vi "Write Control Width.vi"(8 "error in":errorcluster, 10 "Width":u32, 11 "Control in":refnum<vi>) -> (0 "error out":errorcluster, 3 "Control":refnum<vi>)   [LabVIEW 2020, in "VolatusGUIEditorCore.lvlib"]
uses:
  VolatusGUIEditorCore.lvlib
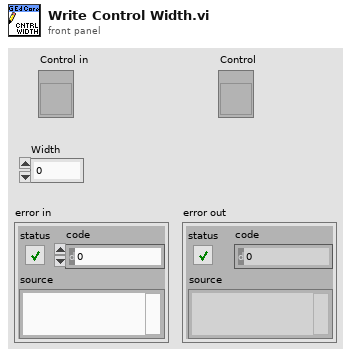
[diagram p1: front panel]
types:
  T1 = typedef "LVBoundsTypeDef.ctl" = cluster{"Width":u32, "Height":u32}
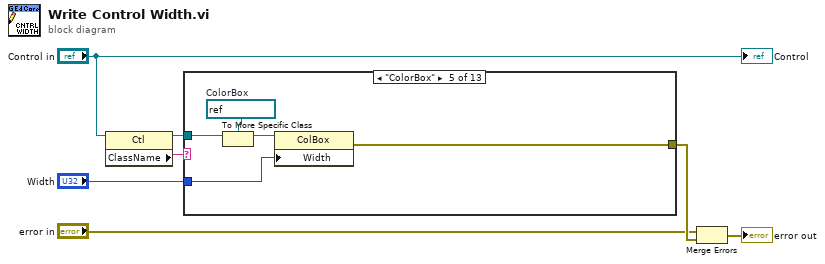
[diagram p0: block diagram]
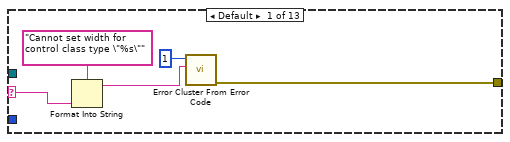
[diagram p2: hidden frame]
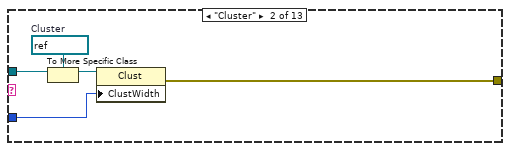
[diagram p3: hidden frame]
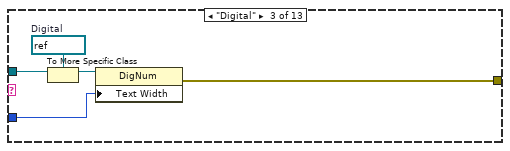
[diagram p4: hidden frame]
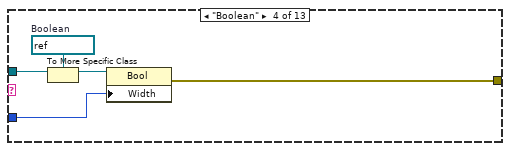
[diagram p5: hidden frame]
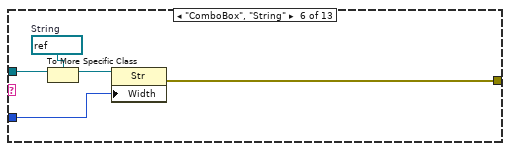
[diagram p6: hidden frame]
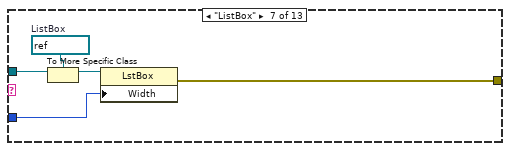
[diagram p7: hidden frame]
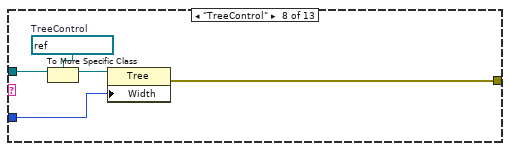
[diagram p8: hidden frame]
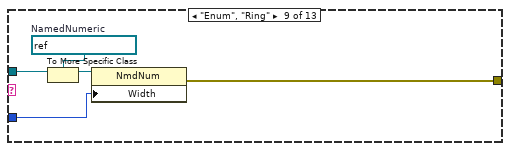
[diagram p9: hidden frame]
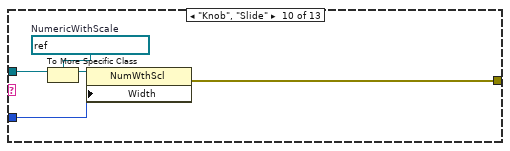
[diagram p10: hidden frame]
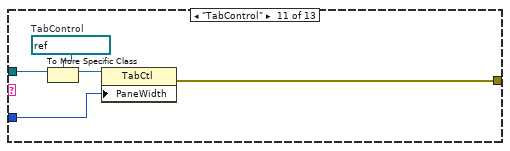
[diagram p11: hidden frame]
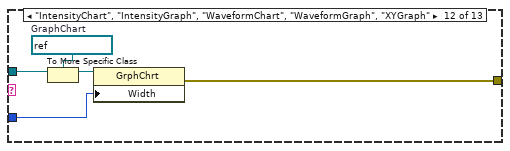
[diagram p12: hidden frame]
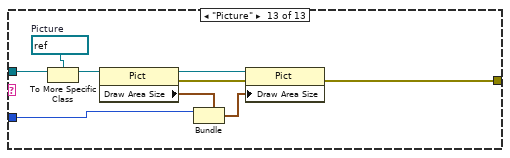
[diagram p13: hidden frame]
diagram:
  n1 = property class="Ctl"(reference="Control in") -> (reference out=w6:refnum<vi>, "ClassName"=w7:string)  [unwired: 1 in, 1 out]
  n2 = case shown="\"ColorBox\"" w7 {
    selector: w7 -> [w9 _ _ _ _ _ _ _ _ _ _ _ _]
    tunnel: w6 -> [_ w17 w22 w27 w32 w37 w42 w47 w52 w57 w62 w67 w76]
    tunnel: "Width" -> [_ w14 w19 w24 w29 w34 w39 w44 w49 w54 w59 w64 w72]
    tunnel: [w12 w13 w18 w23 w28 w33 w38 w43 w48 w53 w58 w63 w68] -> w3
    frame Default {
      n3 = Format Into String(format string="Cannot set width for control class type \"%s\"", w9) -> (resulting string=w8:string)  [unwired: 2 in, 1 out]
      n4 = call <vilib>:"Error Cluster From Error Code.vi"("error message (\"\")"=w8, "error code (0)"=1) -> ("error out"=w12:errorcluster)  [unwired: 7 in]
    }
    frame "Cluster" {
      w16 = refnum<vi> refnum  # Cluster
      n5 = To More Specific Class(target class=w16, reference=w17) -> (specific class reference=w15:refnum<vi>)  [unwired: 1 in, 1 out]
      n6 = property class="Clust"(reference=w15, "ClustWidth"=w14) -> (error out=w13:errorcluster)  [unwired: 1 in, 1 out]
    }
    frame "Digital" {
      w21 = refnum<vi> refnum  # Digital
      n7 = To More Specific Class(target class=w21, reference=w22) -> (specific class reference=w20:refnum<vi>)  [unwired: 1 in, 1 out]
      n8 = property class="DigNum"(reference=w20, "Text Width"=w19) -> (error out=w18:errorcluster)  [unwired: 1 in, 1 out]
    }
    frame "Boolean" {
      w26 = refnum<vi> refnum  # Boolean
      n9 = To More Specific Class(target class=w26, reference=w27) -> (specific class reference=w25:refnum<vi>)  [unwired: 1 in, 1 out]
      n10 = property class="Bool"(reference=w25, "Width"=w24) -> (error out=w23:errorcluster)  [unwired: 1 in, 1 out]
    }
    frame "ColorBox" {
      w31 = refnum<vi> refnum  # ColorBox
      n11 = To More Specific Class(target class=w31, reference=w32) -> (specific class reference=w30:refnum<vi>)  [unwired: 1 in, 1 out]
      n12 = property class="ColBox"(reference=w30, "Width"=w29) -> (error out=w28:errorcluster)  [unwired: 1 in, 1 out]
    }
    frame "ComboBox", "String" {
      w36 = refnum<vi> refnum  # String
      n13 = To More Specific Class(target class=w36, reference=w37) -> (specific class reference=w35:refnum<vi>)  [unwired: 1 in, 1 out]
      n14 = property class="Str"(reference=w35, "Width"=w34) -> (error out=w33:errorcluster)  [unwired: 1 in, 1 out]
    }
    frame "ListBox" {
      w41 = refnum<vi> refnum  # ListBox
      n15 = To More Specific Class(target class=w41, reference=w42) -> (specific class reference=w40:refnum<vi>)  [unwired: 1 in, 1 out]
      n16 = property class="LstBox"(reference=w40, "Width"=w39) -> (error out=w38:errorcluster)  [unwired: 1 in, 1 out]
    }
    frame "TreeControl" {
      w46 = refnum<vi> refnum  # TreeControl
      n17 = To More Specific Class(target class=w46, reference=w47) -> (specific class reference=w45:refnum<vi>)  [unwired: 1 in, 1 out]
      n18 = property class="Tree"(reference=w45, "Width"=w44) -> (error out=w43:errorcluster)  [unwired: 1 in, 1 out]
    }
    frame "Enum", "Ring" {
      w51 = refnum<vi> refnum  # NamedNumeric
      n19 = To More Specific Class(target class=w51, reference=w52) -> (specific class reference=w50:refnum<vi>)  [unwired: 1 in, 1 out]
      n20 = property class="NmdNum"(reference=w50, "Width"=w49) -> (error out=w48:errorcluster)  [unwired: 1 in, 1 out]
    }
    frame "Knob", "Slide" {
      w56 = refnum<vi> refnum  # NumericWithScale
      n21 = To More Specific Class(target class=w56, reference=w57) -> (specific class reference=w55:refnum<vi>)  [unwired: 1 in, 1 out]
      n22 = property class="NumWthScl"(reference=w55, "Width"=w54) -> (error out=w53:errorcluster)  [unwired: 1 in, 1 out]
    }
    frame "TabControl" {
      w61 = refnum<vi> refnum  # TabControl
      n23 = To More Specific Class(target class=w61, reference=w62) -> (specific class reference=w60:refnum<vi>)  [unwired: 1 in, 1 out]
      n24 = property class="TabCtl"(reference=w60, "PaneWidth"=w59) -> (error out=w58:errorcluster)  [unwired: 1 in, 1 out]
    }
    frame "IntensityChart", "IntensityGraph", "WaveformChart", "WaveformGraph", "XYGraph" {
      w66 = refnum<vi> refnum  # GraphChart
      n25 = To More Specific Class(target class=w66, reference=w67) -> (specific class reference=w65:refnum<vi>)  [unwired: 1 in, 1 out]
      n26 = property class="GrphChrt"(reference=w65, "Width"=w64) -> (error out=w63:errorcluster)  [unwired: 1 in, 1 out]
    }
    frame "Picture" {
      w75 = refnum<vi> refnum  # Picture
      n27 = To More Specific Class(target class=w75, reference=w76) -> (specific class reference=w74:refnum<vi>)  [unwired: 1 in, 1 out]
      n28 = property class="Pict"(reference=w74) -> (reference out=w71:refnum<vi>, error out=w69:errorcluster, "Draw Area Size"=w73:T1)  [unwired: 1 in]
      n29 = Bundle(cluster=w73, "Width"=w72) -> (w70:T1)  [unwired: 1 in]
      n30 = property class="Pict"(reference=w71, error in=w69, "Draw Area Size"=w70) -> (error out=w68:errorcluster)  [unwired: 1 out]
    }
  }
  n31 = Merge Errors("error in", w3) -> (→"error out":errorcluster)
  "Control" <- "Control in"
